vi "Write Number of Crossover Points.vi"(8 "error in (no error)":errorcluster, 10 "X-Point":T1, 11 "N-Point Crossover in":refnum<class "N-Point Crossover.lvclass">) -> (0 "error out":errorcluster, 3 "N-Point Crossover out":refnum<class "N-Point Crossover.lvclass">)   [LabVIEW 2016, in "N-Point Crossover.lvclass"]
uses:
  N-Point Crossover.lvclass
  _Typedefs/X-Point Crossover.ctl
  N-Point Crossover.lvclass/N-Point Crossover.ctl
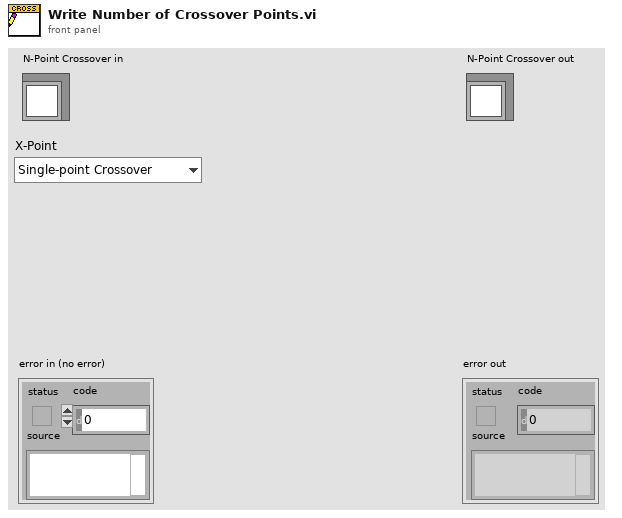
[diagram p1: front panel]
types:
  T1 = typedef "N-Point Crossover.lvclass/X-Point Crossover.ctl" = enum16{"Single-point Crossover", "Dual-point Crossover"}
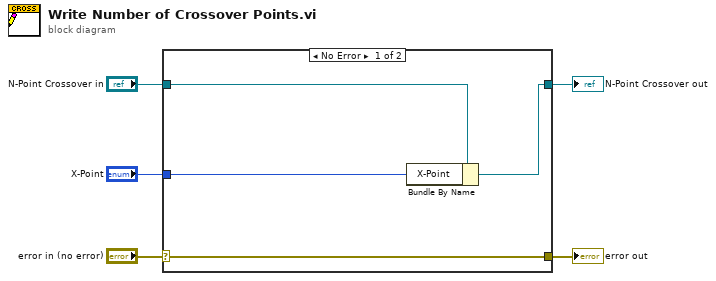
[diagram p0: block diagram]
diagram:
  n1 = case shown="No Error" "error in (no error)" {
    selector: "error in (no error)" -> [w9 w10]
    tunnel: [w9 w10] -> w4
    tunnel: [w7 w11] -> w2
    tunnel: "N-Point Crossover in" -> [w8 w11]
    tunnel: "X-Point" -> [w6 _]
    frame No Error {
      n2 = Bundle By Name(cluster=w8, "X-Point"=w6) -> (w7:refnum<class "N-Point Crossover.lvclass">)
    }
    frame Error {
    }
  }
  "error out" <- w4
  "N-Point Crossover out" <- w2
